vi "Cmd_Q.vi"(7 "VISA resource name":refnum<visa-resource-name>) -> (0 "Position 2":string, 1 "Position 1":string, 2 "Positon 3":string, 3 "Position 4":string, 4 "Status":string, 5 "VISA resource dup":refnum<visa-resource-name>, 6 "OK Done":bool, 8 "Q String":string)   [LabVIEW 2010]
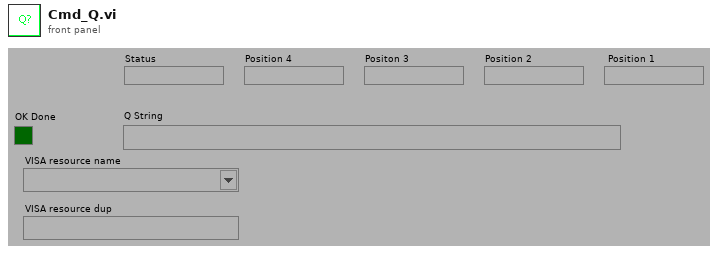
[diagram p1: front panel]
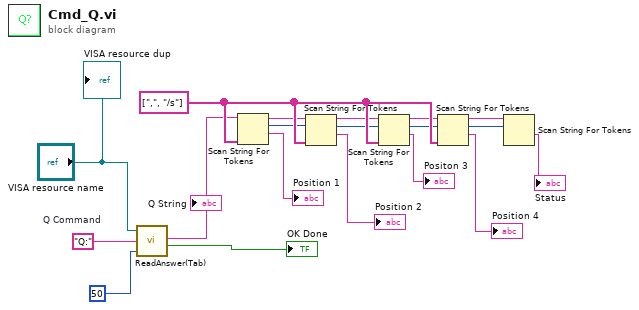
[diagram p0: block diagram]
diagram:
  w1 = "Q:"  # Q Command
  w19 = string[] [",", "/s"] ("delimiters (\\s,\\t,\\r,\\n)")
  n1 = call "ReadAnswer(Tab).vi"("Bytes to Read"=u32 50, "Command (\\r is appended)"=w1, "VRN IN"="VISA resource name") -> ("OKdone"=→"OK Done":bool, "String Received"=w4:string)  [unwired: 2 out]
  "Q String" <- w4
  n2 = Scan String For Tokens(6:w19, 9:w4) -> (1:→"Position 1":string, 2:w6:i32, 3:w7:string)  [unwired: 4 in, 1 out]
  n3 = Scan String For Tokens(6:w19, 8:w6, 9:w7) -> (1:→"Position 2":string, 2:w10:i32, 3:w9:string)  [unwired: 3 in, 1 out]
  n4 = Scan String For Tokens(6:w19, 8:w10, 9:w9) -> (1:→"Positon 3":string, 2:w12:i32, 3:w11:string)  [unwired: 3 in, 1 out]
  n5 = Scan String For Tokens(6:w19, 8:w12, 9:w11) -> (1:→"Position 4":string, 2:w14:i32, 3:w13:string)  [unwired: 3 in, 1 out]
  n6 = Scan String For Tokens(8:w14, 9:w13) -> (1:→"Status":string)  [unwired: 4 in, 3 out]
  "VISA resource dup" <- "VISA resource name"
